vi "Register AI IRQ.vi"(4 "Callback VI Reference":T1, 6 "Threshold":dbl=2.5, 8 "error in (no error)":errorcluster, 9 "Analog Interrupt Type":T2, 10 "Channel Name":tag, 11 "IRQ Number":u8) -> (0 "error out":errorcluster)   [LabVIEW 2021, in "IO IRQ.lvlib"]
uses:
  <vilib>/myRIO/Instrument Drivers/IRQ/IO IRQ/IO IRQ.lvlib
  <vilib>/myRIO/Instrument Drivers/IRQ/IO IRQ/vis/myRIO Register AI IRQ.xnode
  <vilib>/myRIO/Common/Instrument Driver Framework/myRIO v1.0/IRQ/typedefs/Callback VI Ref.ctl
  <vilib>/myRIO/Common/Instrument Driver Framework/myRIO v1.0/IRQ/typedefs/AI IRQ Type.ctl
  <vilib>/userdefined/High Color/nirio_resource_hc.ctl
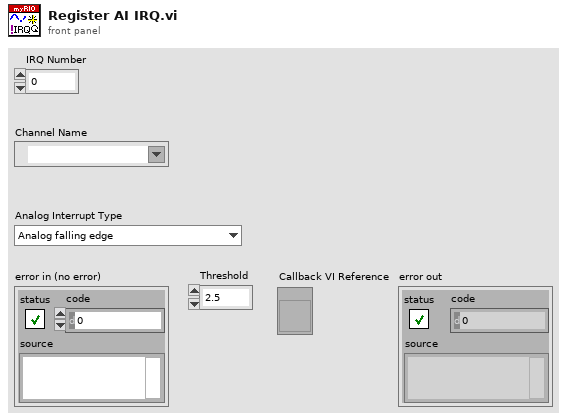
[diagram p1: front panel]
types:
  T1 = typedef "Callback VI Ref.ctl" = refnum<vi>
  T2 = typedef "AI IRQ Type.ctl" = enum16{"Analog falling edge", "Analog rising edge"}
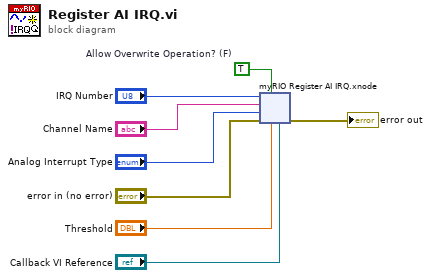
[diagram p0: block diagram]
diagram:
  w4 = TRUE  # Allow Overwrite Operation? (F)
  n1 = xnode "myRIO Register AI IRQ.xnode"("error in (no error)"="error in (no error)", "Channel Name"="Channel Name", "Callback VI Reference"="Callback VI Reference", "Allow Overwrite Operation? (F)"=w4, "Threshold"="Threshold", "IRQ Number"="IRQ Number", "Analog Interrupt Type"="Analog Interrupt Type") -> ("error out"=→"error out":errorcluster)  [unwired: 1 in]
